vi "Projeto A - Sistema Eletrocardiográfico - LabVIEW.vi"() -> ()   [LabVIEW 2021]
panel:
  out "BPM":dbl
  out "Pacemaker":bool
  out "Atropina":bool
  out "Propanolol":bool
  in  "Save Button":bool
  out "BPM":dbl(knob) scale=0.0..200.0
  out "Desfibrilhador":bool
  in  "VISA resource name":refnum<visa-resource-name>
  out "R Wave":bool
  in  "Stop Button":bool
  in  "Upper Limit":dbl
  in  "Lower Limit":dbl
  in  "Sampling Rate":u16(ring) items=["25 S/s", "50 S/s", "100 S/s", "200 S/s", "Aquisition Stopped"]
  out "Waveform Chart":u8(graph)
  out "error out":errorcluster
  in  "error in":errorcluster
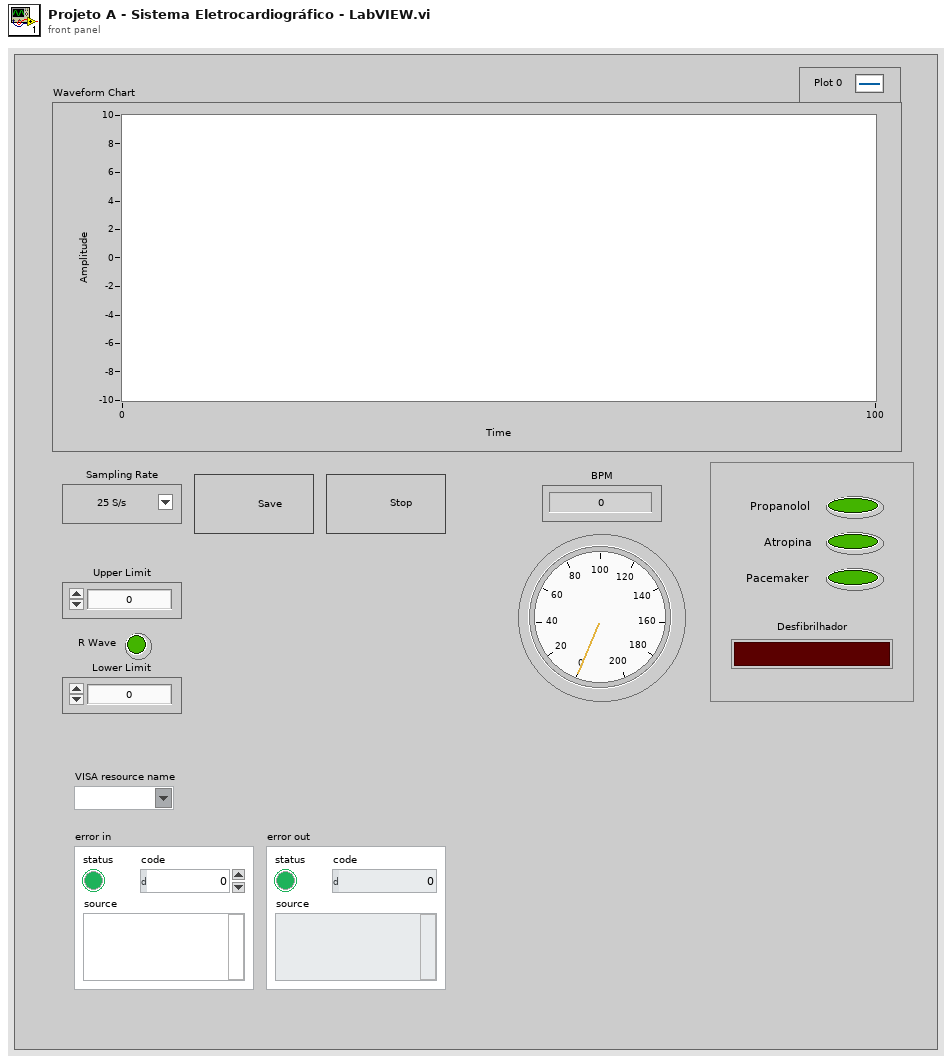
[diagram p1: front panel]
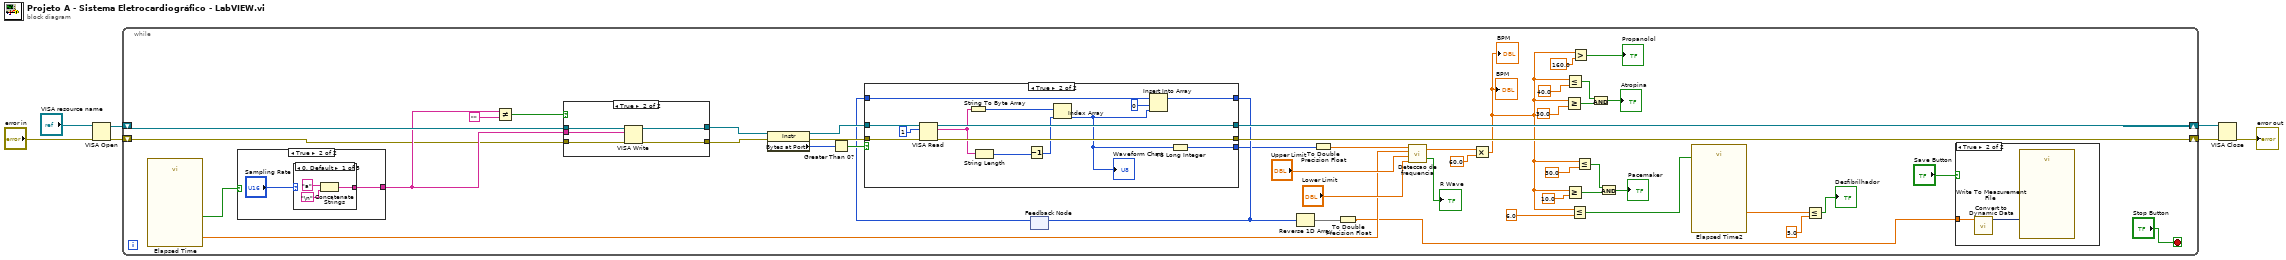
[diagram p0: block diagram]
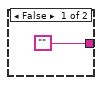
[diagram p2: hidden frame]
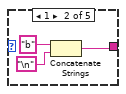
[diagram p3: hidden frame]
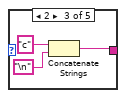
[diagram p4: hidden frame]
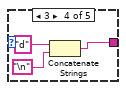
[diagram p5: hidden frame]
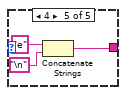
[diagram p6: hidden frame]
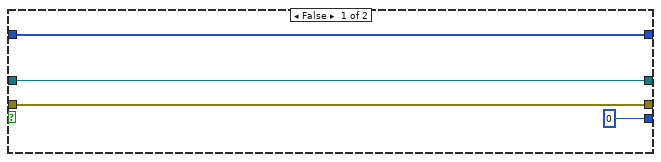
[diagram p8: hidden frame]
diagram:
  n1 = VISA Open(error in (no error)="error in", VISA resource name="VISA resource name") -> (VISA resource name=w5:refnum<visa-resource-name>, error out=w4:errorcluster)  [unwired: 3 in]
  n2 = while {
    shift-right: [w48] -> w3
    shift-left: w5 -> [w53]
    shift-right: [w47] -> w2
    shift-left: w4 -> [w11]
    stop <- "Stop Button" stop-if-true
    n3 = call "Elapsed Time"() -> ("Present (s)"=w15:dbl, "Time has Elapsed"=w35:bool)  [unwired: 12 in, 6 out]
    n4 = case shown="True" w35 {
      tunnel: ["" w55] -> w19
      frame False {
      }
      frame True {
        n5 = case shown="0, Default" "Sampling Rate" {
          tunnel: [w57 w60 w63 w66 w69] -> w55
          frame 0, Default {
            n6 = Concatenate Strings("a", "\n") -> (w57:string)
          }
          frame 1 {
            n7 = Concatenate Strings("b", "\n") -> (w60:string)
          }
          frame 2 {
            n8 = Concatenate Strings("c", "\n") -> (w63:string)
          }
          frame 3 {
            n9 = Concatenate Strings("d", "\n") -> (w66:string)
          }
          frame 4 {
            n10 = Concatenate Strings("e", "\n") -> (w69:string)
          }
        }
      }
    }
    n11 = Not Equal?(x=w19, y="") -> (x != y?=w18:bool)
    n12 = case shown="True" w18 {
      tunnel: w53 -> [w93 w98]
      tunnel: w11 -> [w92 w97]
      tunnel: [w93 w96] -> w52
      tunnel: [w92 w95] -> w51
      tunnel: w19 -> [_ w94]
      frame False {
      }
      frame True {
        n13 = VISA Write(VISA resource name=w98, write buffer=w94, error in (no error)=w97) -> (VISA resource name out=w96:refnum<visa-resource-name>, error out=w95:errorcluster)  [unwired: 1 out]
      }
    }
    n14 = property class="Instr"(reference=w52, error in=w51) -> (reference out=w50:refnum<visa-resource-name>, error out=w49:errorcluster, "Bytes at Port"=w45:u32)
    n15 = Greater Than 0?(x=w45) -> (x > 0?=w44:bool)
    n16 = feedback #1() -> (w43:u8[])  [unwired: 1 in]
    n17 = case shown="True" w44 {
      tunnel: w50 -> [w77 w91]
      tunnel: w49 -> [w76 w90]
      tunnel: [w77 w89] -> w48
      tunnel: [w76 w88] -> w47
      tunnel: w43 -> [w75 w85]
      tunnel: [w75 w84] -> w40
      tunnel: [0 w78] -> w38
      frame False {
      }
      frame True {
        n18 = VISA Read(VISA resource name=w91, byte count=u32 1, error in (no error)=w90) -> (VISA resource name out=w89:refnum<visa-resource-name>, read buffer=w82:string, error out=w88:errorcluster)  [unwired: 1 out]
        n19 = String To Byte Array(string=w82) -> (unsigned byte array=w83:u8[])
        n20 = String Length(string=w82) -> (length=w81:i32)
        n21 = Decrement(x=w81) -> (x-1=w80:i32)
        n22 = Index Array(array=w83, index=w80) -> (element=w79:u8)
        "Waveform Chart" <- w79
        n23 = Insert Into Array(array=w85, index=0, new element=w79) -> (w84:u8[])
        n24 = To Long Integer(number=w79) -> (32bit integer=w78:i32)
      }
    }
    n25 = feedback-in #1(w40) -> ()
    n26 = Reverse 1D Array(array=w40) -> (reversed array=w41:u8[])
    n27 = To Double Precision Float(number=w38) -> (double precision float=w39:dbl)
    n28 = To Double Precision Float(number=w41) -> (double precision float=w8:dbl[])
    n29 = call "Deteccao de frequencia.vi"("Limiar inferior de deteccao"="Lower Limit", "Limiar superior de deteccao"="Upper Limit", "Tempo (s)"=w15, "Medida do sinal"=w39) -> ("Deteccao de limiar"=→"R Wave":bool, "Frequencia (Hz)"=w33:dbl)
    n30 = Multiply(x=w33, y=60.0) -> (x*y=w9:dbl)
    "BPM" <- w9
    "BPM" <- w9
    n31 = Greater Or Equal?(x=w9, y=30.0) -> (x >= y?=w24:bool)
    n32 = Less Or Equal?(x=w9, y=40.0) -> (x <= y?=w25:bool)
    n33 = Greater Or Equal?(x=w9, y=10.0) -> (x >= y?=w22:bool)
    n34 = Less Or Equal?(x=w9, y=6.0) -> (x <= y?=w16:bool)
    n35 = Greater?(x=w9, y=160.0) -> (0:→"Propanolol":bool)
    n36 = Less Or Equal?(x=w9, y=30.0) -> (x <= y?=w23:bool)
    n37 = And(x=w25, y=w24) -> (x .and. y?=→"Atropina":bool)
    n38 = And(x=w23, y=w22) -> (x .and. y?=→"Pacemaker":bool)
    n39 = call "Elapsed Time2"("Reset"=w16) -> ("Elapsed Time (s)"=w14:dbl)  [unwired: 11 in, 7 out]
    n40 = Less Or Equal?(x=w14, y=5.0) -> (x <= y?=→"Desfibrilhador":bool)
    n41 = case shown="True" "Save Button" {
      tunnel: w8 -> [_ w72]
      frame False {
      }
      frame True {
        n42 = call "Convert to Dynamic Data"("Array"=w72) -> ("Dynamic Data Type"=w73:dynamicdata)  [unwired: 3 in]
        n43 = call "Write To Measurement File"("Signals"=w73) -> ()  [unwired: 16 in, 3 out]
      }
    }
  }
  n44 = VISA Close(VISA resource name=w3, error in (no error)=w2) -> (error out=→"error out":errorcluster)
